vi "NTU Read Pin Map.vi"(8 "error in (no error)":errorcluster, 11 "I-O in":refnum<class "Copy of I-O.lvclass">) -> (0 "error out":errorcluster, 2 "Pin Map":T1={"Region Valves"=[49, 52, 0, 0], "Extra Valves"=[[0.0, 48.0, 0.0, 0.0, 0.0]], "Tool Primary Valve"=51, "Tool Secondary Valve"=50, "Region Sensors"=[37, 41, 37], "Extra Sensors"=[[36.0, 37.0, 0.0, 0.0]], "Tool Primary Sensor"=39.0, "Tool Secondary Sensor"=38.0, "Compression Sensor"=31.0, "5V"=50, "NTU_Glue"=0.0}, 3 "I-O out":refnum<class "Copy of I-O.lvclass">)   [LabVIEW 2016]
uses:
  Copy of I-O.lvclass
  D:/INTT/Classes/Controllers/Copy of Controller Folder/Copy of Controller.lvclass
  Pin Map.ctl
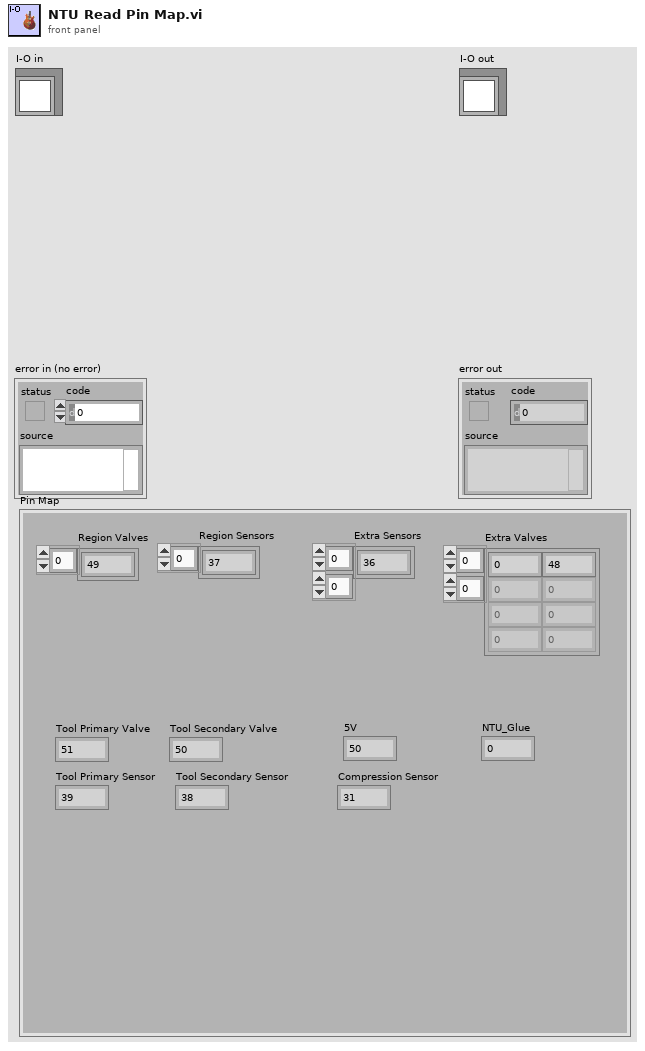
[diagram p1: front panel]
types:
  T1 = typedef "Copy of I-O.lvclass/Pin Map.ctl" = cluster{"Region Valves":i32[], "Extra Valves":dbl[][], "Tool Primary Valve":i32, "Tool Secondary Valve":i32, "Region Sensors":i32[], "Extra Sensors":dbl[][], "Tool Primary Sensor":dbl, "Tool Secondary Sensor":dbl, "Compression Sensor":dbl, "5V":i32, "NTU_Glue":dbl}
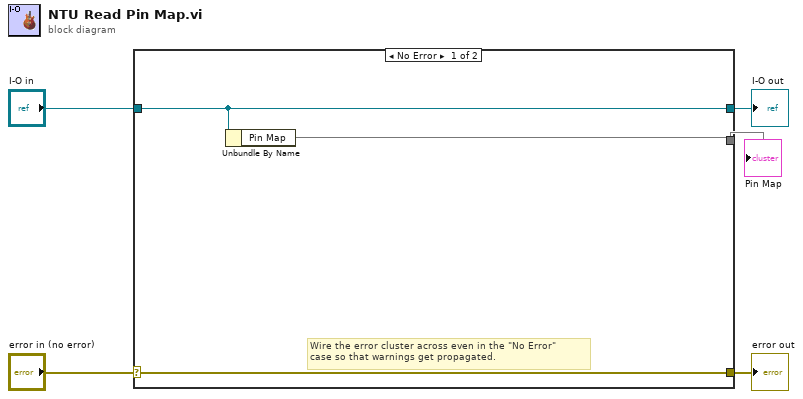
[diagram p0: block diagram]
diagram:
  n1 = case shown="No Error" "error in (no error)" {
    selector: "error in (no error)" -> [w8 w10]
    tunnel: [w8 w10] -> w4
    tunnel: [w7 w9] -> w2
    tunnel: "I-O in" -> [w7 w9]
    tunnel: [w6 _] -> w1
    frame No Error {
      # "Wire the error cluster across even in the \"No Error\"\ncase so that warnings get propagated."
      n2 = Unbundle By Name(w7) -> ("Pin Map"=w6)
    }
    frame Error {
    }
  }
  "error out" <- w4
  "I-O out" <- w2
  "Pin Map" <- w1
